vi "OpenY16DeviceByXML.vi"(2 "error in (no error)":errorcluster, 3 "Filename":string, 4 "ICImagingControl":refnum<k7>) -> (0 "error out":errorcluster, 1 "ICImagingControl 2":refnum<k7>)   [LabVIEW 2010]
doc: "This VI is for handling Y16 sink (pixelformat) only.\nOpen a camera using a previously created XML file. Create the XML with the DeviceXMLGenerator.exe in tne samples\\DeviceXMLGenerator directory.The OverlayBitmap is disabled."
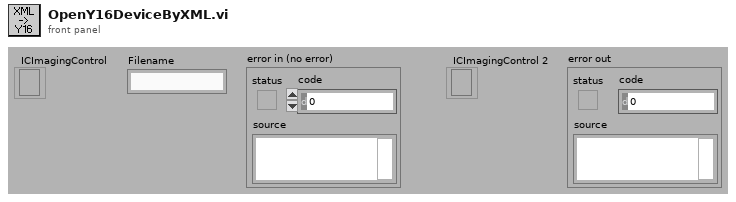
[diagram p1: front panel]
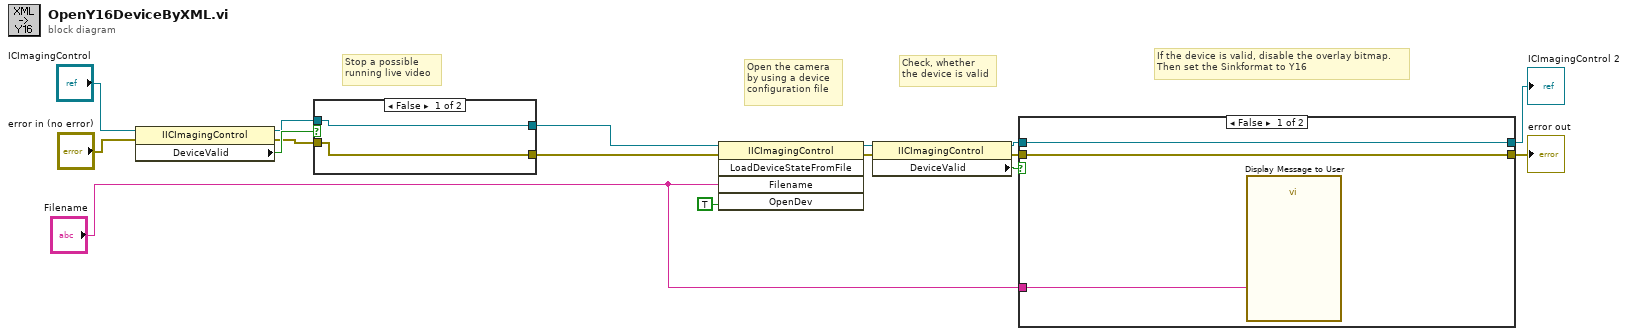
[diagram p0: block diagram]
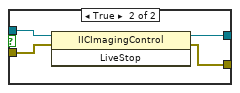
[diagram p2: hidden frame]
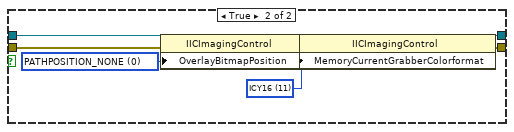
[diagram p3: hidden frame]
diagram:
  # "If the device is valid, disable the overlay bitmap.\nThen set the Sinkformat to Y16"
  # "Check, whether\nthe device is valid"
  # "Open the camera\nby using a device \nconfiguration file"
  # "Stop a possible\nrunning live video"
  n1 = property class="IICImagingControl"(reference="ICImagingControl", error in="error in (no error)") -> (reference out=w4:refnum<k7>, error out=w3:errorcluster, "DeviceValid"=w5:bool)
  n2 = case shown="False" w5 {
    tunnel: w4 -> [w18 w22]
    tunnel: w3 -> [w17 w21]
    tunnel: [w17 w20] -> w2
    tunnel: [w18 w19] -> w1
    frame False {
    }
    frame True {
      n3 = invoke class="IICImagingControl" method="LiveStop"(reference=w22, error in=w21) -> (reference out=w19:refnum<k7>, error out=w20:errorcluster)  [unwired: 1 in, 1 out]
    }
  }
  n4 = invoke class="IICImagingControl" method="LoadDeviceStateFromFile"(reference=w1, error in=w2, "Filename"="Filename", "OpenDev"=TRUE) -> (reference out=w11:refnum<k7>, error out=w8:errorcluster)  [unwired: 1 in, 3 out]
  n5 = property class="IICImagingControl"(reference=w11, error in=w8) -> (reference out=w13:refnum<k7>, error out=w14:errorcluster, "DeviceValid"=w12:bool)
  n6 = case shown="False" w12 {
    tunnel: w13 -> [w25 w32]
    tunnel: [w25 w29] -> w15
    tunnel: w14 -> [w24 w28]
    tunnel: [w24 w26] -> w16
    tunnel: "Filename" -> [w23 _]
    frame False {
      n7 = call "Display Message to User"("Message"=w23) -> ()  [unwired: 9 in, 2 out]
    }
    frame True {
      w30 = 11 items=["ICRGB32"=1, "ICRGB24"=2, "ICRGB565"=3, "ICRGB555"=4, "ICY8"=5, "ICUYVY"=6, "ICY800"=7, "ICYGB1"=8, "ICYGB0"=9, "ICBY8"=10, "ICY16"=11] ("MemoryCurrentGrabberColorformat")
      w33 = 0 items=["PATHPOSITION_NONE"=0, "PATHPOSITION_DEVICE"=1, "PATHPOSITION_SINK"=2, "PATHPOSITION_DISPLAY"=4] ("OverlayBitmapPosition")
      n8 = property class="IICImagingControl"(reference=w32, error in=w28, "OverlayBitmapPosition"=w33) -> (reference out=w31:refnum<k7>, error out=w27:errorcluster)
      n9 = property class="IICImagingControl"(reference=w31, error in=w27, "MemoryCurrentGrabberColorformat"=w30) -> (reference out=w29:refnum<k7>, error out=w26:errorcluster)
    }
  }
  "error out" <- w16
  "ICImagingControl 2" <- w15
